vi "XMLRelult_Save_To_File.vi"(10 "UUT OUT Data":string[][](array[string]), 11 "XML File Path":path caption="XML文件路径") -> (1 "连接的字符串":string, 2 "字符串":string, 3 "XML File Path(duplicate)":path caption="XML文件路径（副本）")   [LabVIEW 2018]
uses:
  Subvi/Global.vi
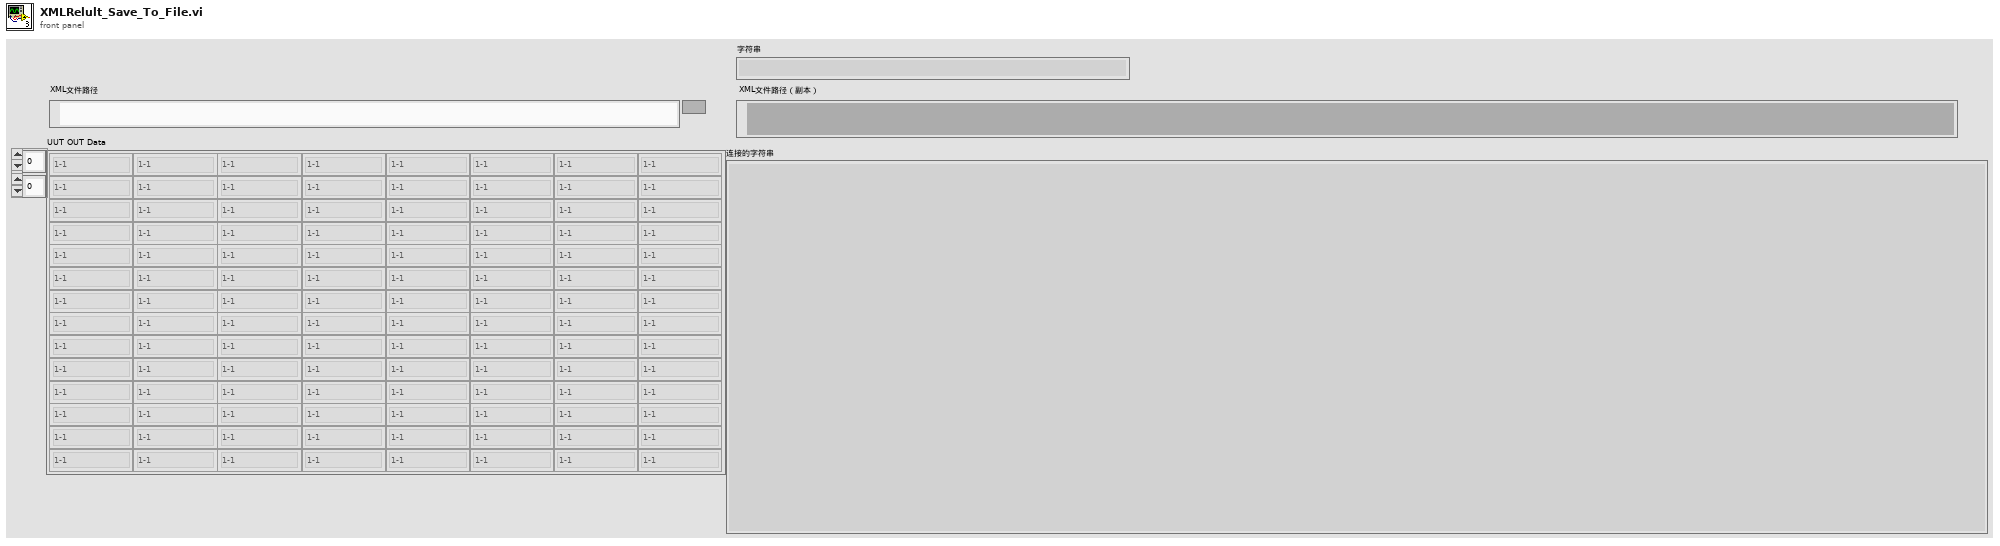
[diagram p1: front panel]
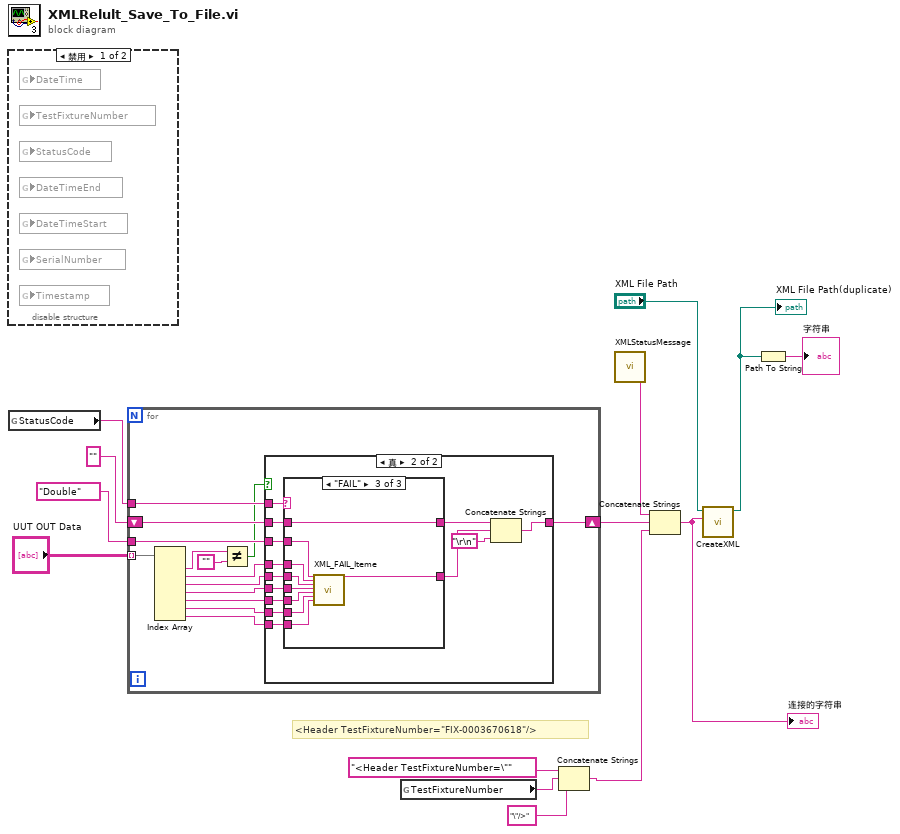
[diagram p0: block diagram]
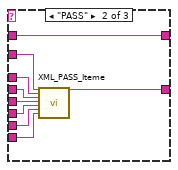
[diagram p4: hidden frame]
diagram:
  # "<Header TestFixtureNumber=\"FIX-0003670618\"/>"
  n1 = disable-structure shown="禁用" {
    frame Disabled {
      n2 = global read "Global.vi" "DateTime"() -> ()  [unwired: 1 in]
      n3 = global read "Global.vi" "TestFixtureNumber"() -> ()  [unwired: 1 in]
      n4 = global read "Global.vi" "StatusCode"() -> ()  [unwired: 1 in]
      n5 = global read "Global.vi" "DateTimeEnd"() -> ()  [unwired: 1 in]
      n6 = global read "Global.vi" "DateTimeStart"() -> ()  [unwired: 1 in]
      n7 = global read "Global.vi" "SerialNumber"() -> ()  [unwired: 1 in]
      n8 = global read "Global.vi" "Timestamp"() -> ()  [unwired: 1 in]
    }
    frame Enabled {
    }
  }
  n9 = global read "Global.vi" "StatusCode"() -> (w12:string)
  n10 = for {
    tunnel: w12 -> [w27]
    shift-right: [w25] -> w13
    shift-left: "" -> [w28]
    tunnel: "Double" ("组合框") -> [w26]
    tunnel: "UUT OUT Data" -> [w21] mode=indexing
    n11 = Index Array(array=w21) -> (element #1=w22:string, element #2=w20:string, element #3=w19:string, element #4=w18:string, element #5=w17:string, element #6=w16:string, element #7=w15:string)  [unwired: 7 in]
    n12 = Not Equal?(x=w22, y="") -> (x != y?=w23:bool)
    n13 = case shown="真" w23 {
      tunnel: w28 -> [w29 w42]
      tunnel: w27 -> [_ w41]
      tunnel: w26 -> [_ w40]
      tunnel: [w29 w36] -> w25
      tunnel: w20 -> [_ w35]
      tunnel: w19 -> [_ w34]
      tunnel: w18 -> [_ w33]
      tunnel: w17 -> [_ w32]
      tunnel: w16 -> [_ w31]
      tunnel: w15 -> [_ w30]
      frame False {
      }
      frame True {
        n14 = case shown="\"FAIL\"" w41 {
          tunnel: w42 -> [w43 w50 w59]
          tunnel: [_ w52 w61] -> w38
          tunnel: w40 -> [_ w51 w60]
          tunnel: [w43 w50 w59] -> w37
          tunnel: w35 -> [_ w49 w58]
          tunnel: w34 -> [_ w48 w57]
          tunnel: w33 -> [_ w47 w56]
          tunnel: w32 -> [_ w46 w55]
          tunnel: w31 -> [_ w45 w54]
          tunnel: w30 -> [_ w44 w53]
          frame "假", Default {
          }
          frame "PASS" {
            n15 = call "XML_PASS_Iteme.vi"("组合框"=w51, "Name"=w49, "UpperLimit"=w48, "Value"=w47, "LowerLimit"=w46, "MeasurementUnit"=w45, "StatusCode"=w44) -> ("连接的字符串"=w52:string)  [unwired: 20 in]
          }
          frame "FAIL" {
            n16 = call "XML_FAIL_Iteme.vi"("组合框"=w60, "Name"=w58, "UpperLimit"=w57, "Value"=w56, "LowerLimit"=w55, "MeasurementUnit"=w54, "StatusCode"=w53) -> ("连接的字符串"=w61:string)  [unwired: 20 in]
          }
        }
        n17 = Concatenate Strings(w37, w38, "\r\n") -> (w36:string)
      }
    }
  }
  n18 = global read "Global.vi" "TestFixtureNumber"() -> (w5:string)
  n19 = Concatenate Strings("<Header TestFixtureNumber=\"", w5, "\"/>") -> (w3:string)
  n20 = call "XMLStatusMessage.vi"() -> ("连接的字符串"=w14:string)  [unwired: 10 in, 1 out]
  n21 = Concatenate Strings(w14, w13, w3) -> (w8:string)
  "连接的字符串" <- w8
  n22 = call "CreateXML.vi"("XML Input"=w8, "XML File Path"="XML File Path") -> ("XML File Path(duplicate)"=w2:path)  [unwired: 7 in, 2 out]
  "XML File Path(duplicate)" <- w2
  n23 = Path To String(path=w2) -> (string=→"字符串":string)
